vi "Helium Test - Step 5.vi"(7 "Step":i32, 8 "error in":errorcluster, 9 "Test Results In":T9, 10 "Gas":T8, 11 "Test Configuration":T1) -> (0 "error out":errorcluster, 1 "Test Results Out":T9, 2 "Gas Out":T8 caption="Gas", 3 "Test Configuration Out":T1)   [LabVIEW 2015]
uses:
  CAN Communication/PAS/Typedefs/Session Handle.ctl
  CAN Communication/PAS/PAS.lvclass
  Controls/Test Results.ctl
  Controls/Step Result.ctl
  Controls/Test Configuration.ctl
  Controls/Vacuum Test.ctl
  Controls/Test Timing.ctl
  Controls/Vaccum Thresholds.ctl
  Controls/Helium Test.ctl
  Controls/Helium Thresholds.ctl
  Controls/Functional Test.ctl
  CAN Communication/PAS/Typedefs/Valves.ctl
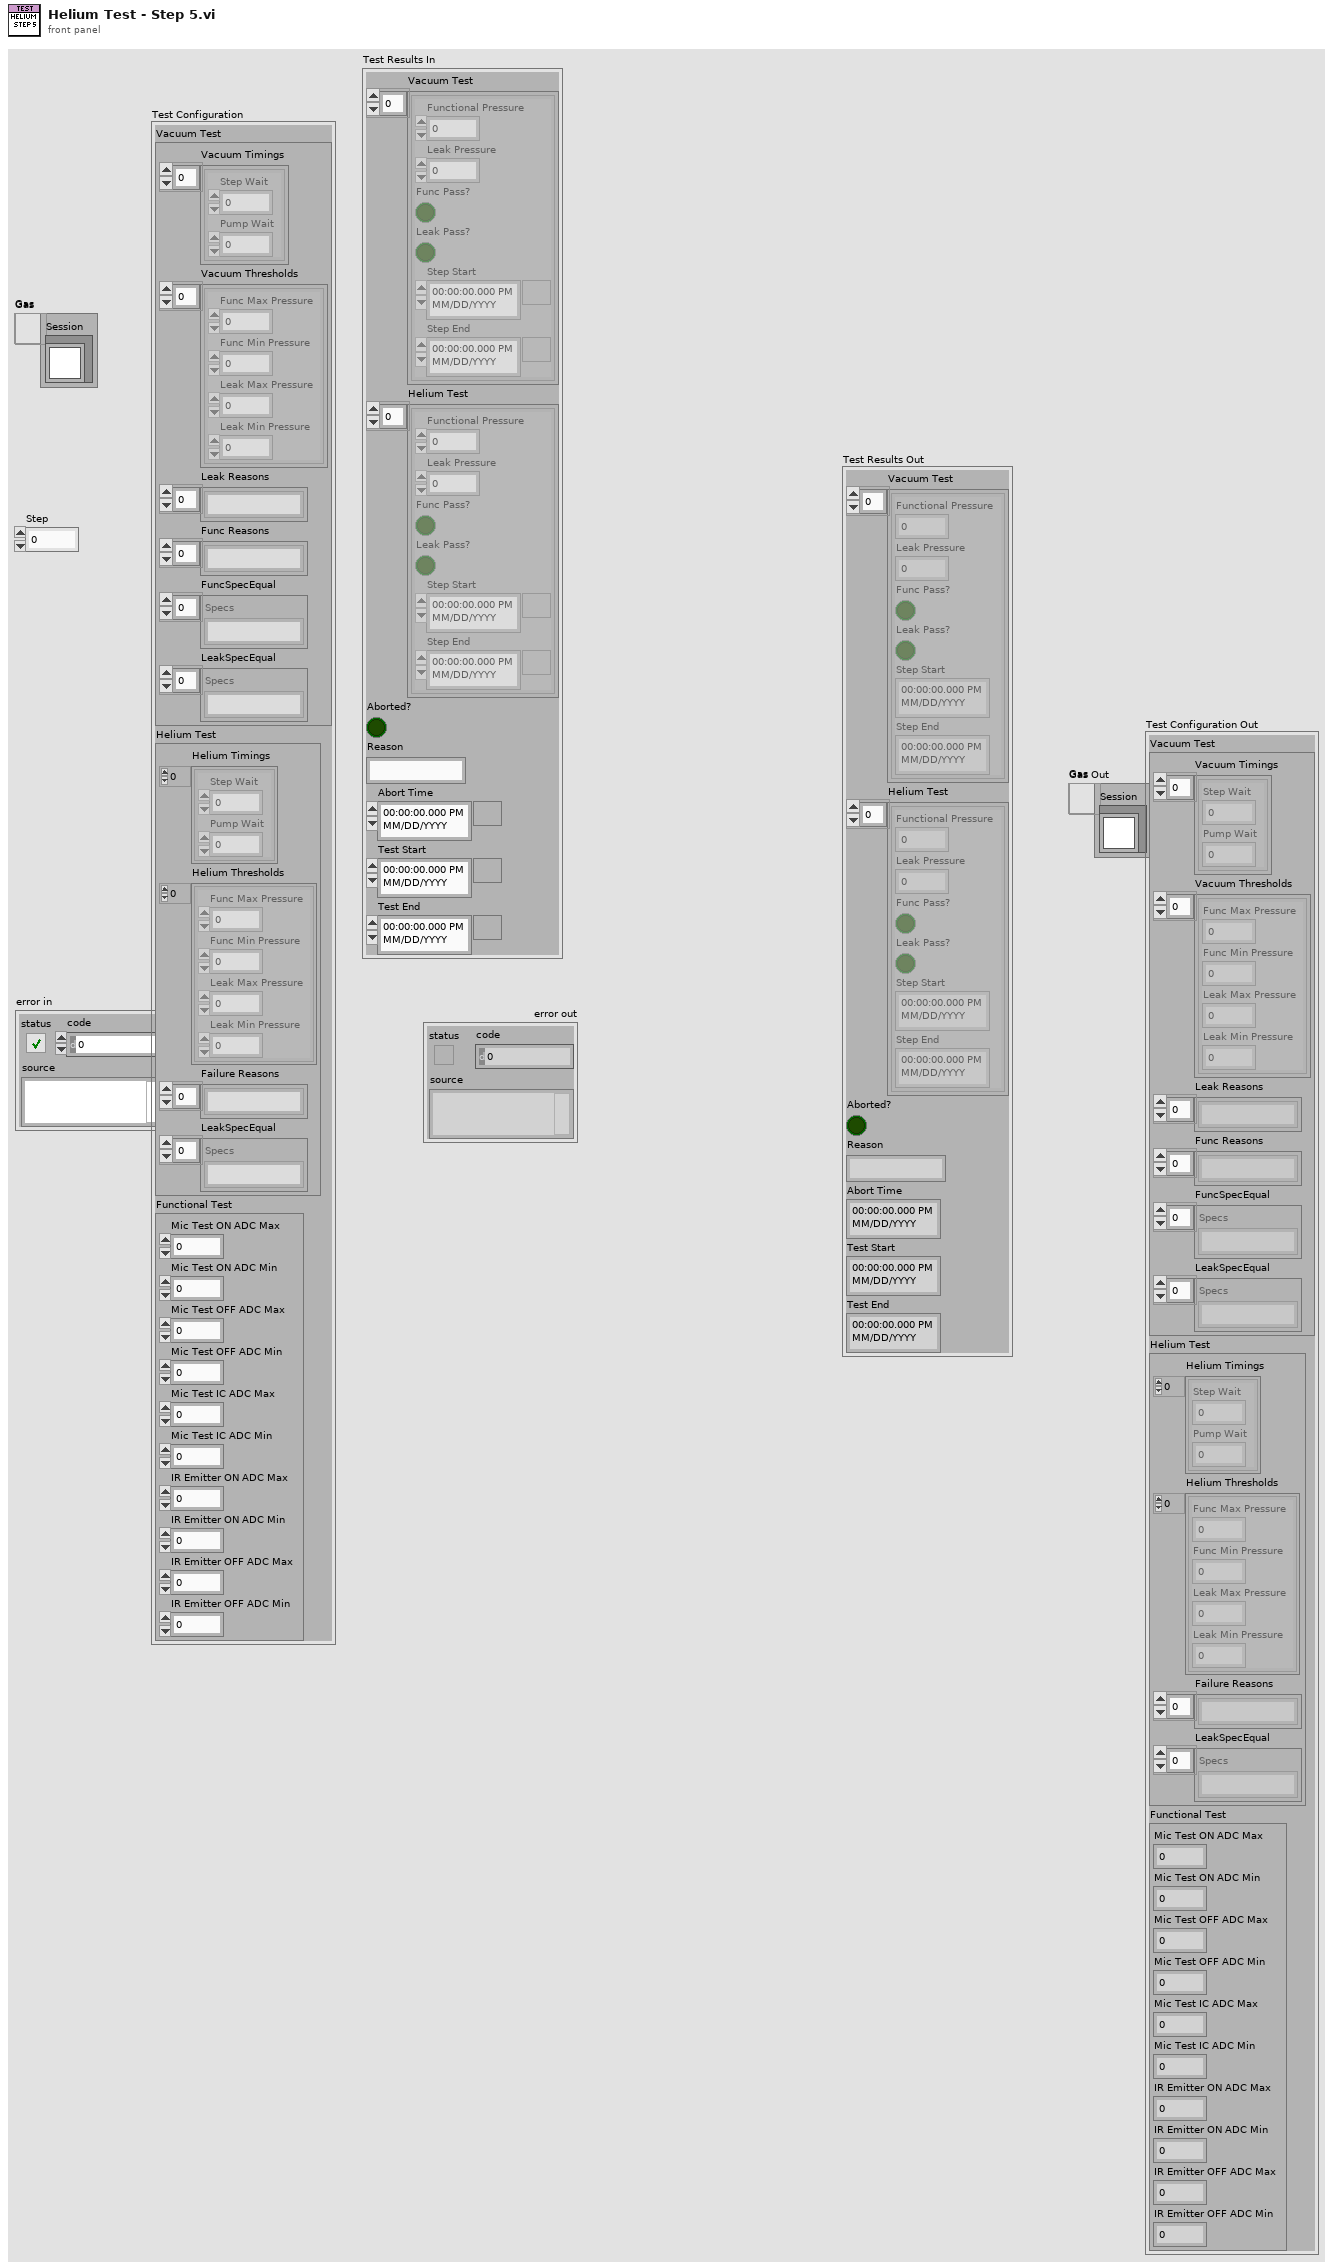
[diagram p1: front panel]
types:
  T1 = typedef "Test Configuration.ctl" = cluster{"Vacuum Test":T2, "Helium Test":T5, "Functional Test":T7}
  T2 = typedef "Vacuum Test.ctl" = cluster{"Vacuum Timings":T3[], "Vacuum Thresholds":T4[], "Leak Reasons":string[], "Func Reasons":string[], "FuncSpecEqual":string[], "LeakSpecEqual":string[]}
  T3 = typedef "Test Timing.ctl" = cluster{"Step Wait":dbl, "Pump Wait":dbl}
  T4 = typedef "Vaccum Thresholds.ctl" = cluster{"Func Max Pressure":dbl, "Func Min Pressure":dbl, "Leak Max Pressure":dbl, "Leak Min Pressure":dbl}
  T5 = typedef "Helium Test.ctl" = cluster{"Helium Timings":T3[], "Helium Thresholds":T6[], "Failure Reasons":string[], "LeakSpecEqual":string[]}
  T6 = typedef "Helium Thresholds.ctl" = cluster{"Func Max Pressure":dbl, "Func Min Pressure":dbl, "Leak Max Pressure":dbl, "Leak Min Pressure":dbl}
  T7 = typedef "Functional Test.ctl" = cluster{"Mic Test ON ADC Max":dbl, "Mic Test ON ADC Min":dbl, "Mic Test OFF ADC Max":dbl, "Mic Test OFF ADC Min":dbl, "Mic Test IC ADC Max":dbl, "Mic Test IC ADC Min":dbl, "IR Emitter ON ADC Max":dbl, "IR Emitter ON ADC Min":dbl, "IR Emitter OFF ADC Max":dbl, "IR Emitter OFF ADC Min":dbl}
  T8 = typedef "PAS.lvclass/Session Handle.ctl" = refnum<data-value>
  T9 = typedef "Test Results.ctl" = cluster{"Vacuum Test":T10[], "Helium Test":T10[], "Aborted?":bool, "Reason":string, "Abort Time":timestamp, "Test Start":timestamp, "Test End":timestamp}
  T10 = typedef "Step Result.ctl" = cluster{"Functional Pressure":dbl, "Leak Pressure":dbl, "Func Pass?":bool, "Leak Pass?":bool, "Step Start":timestamp, "Step End":timestamp}
  T11 = typedef "PAS.lvclass/Valves.ctl" = u16
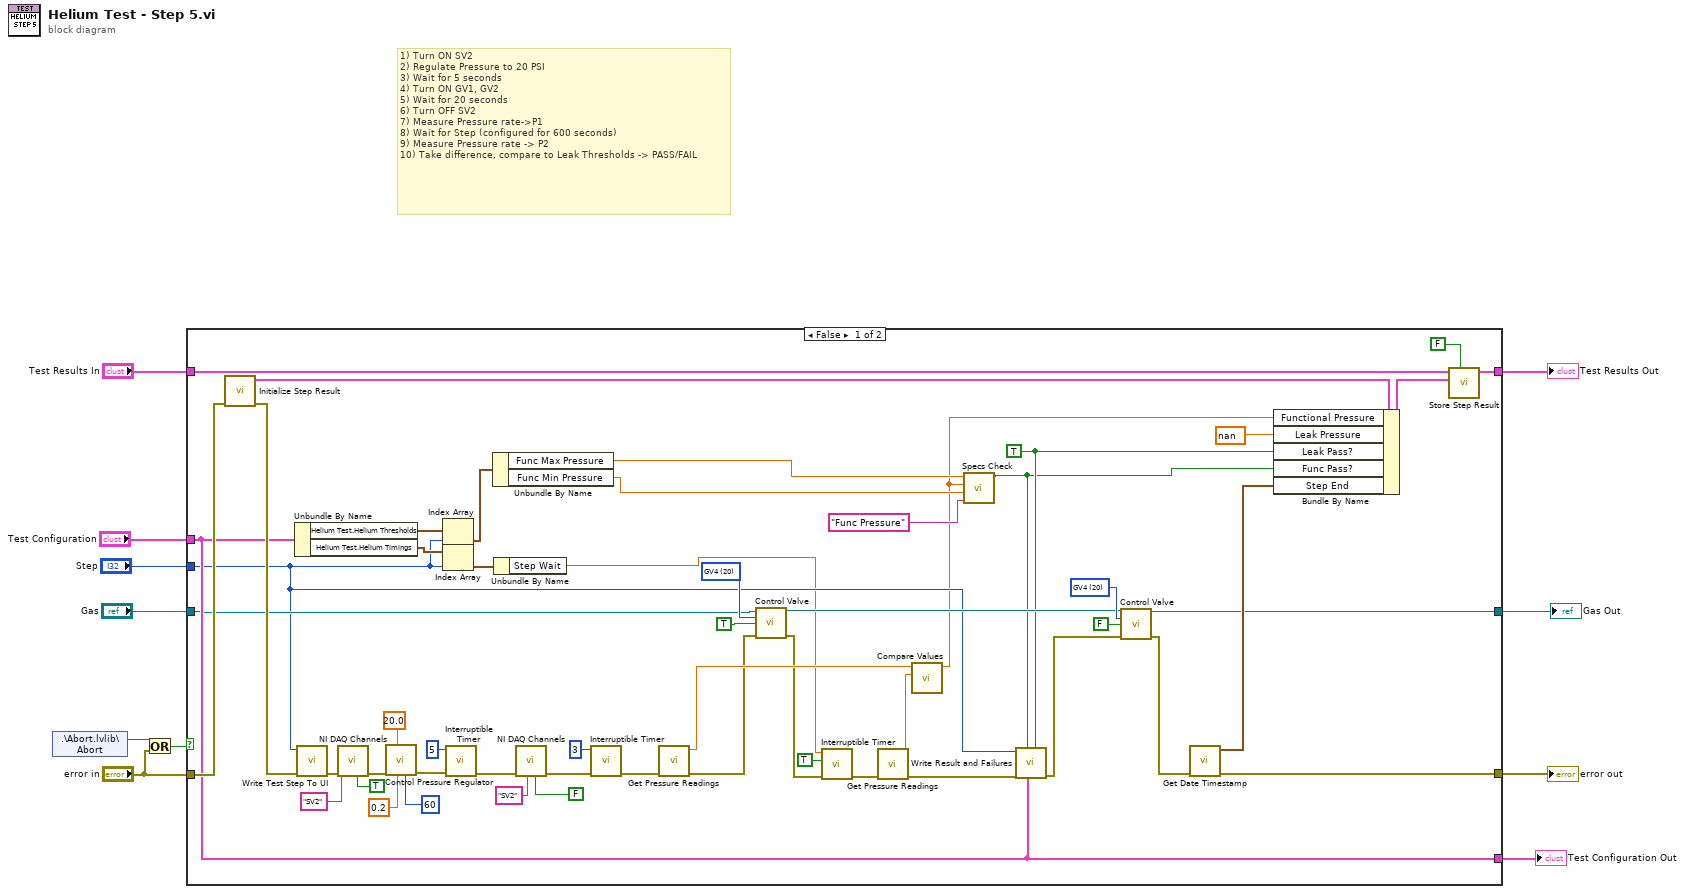
[diagram p0: block diagram]
diagram:
  # "1) Turn ON SV2\n2) Regulate Pressure to 20 PSI\n3) Wait for 5 seconds\n4) Turn ON GV1, GV2\n5) Wait for 20 seconds\n6) Turn OFF SV2\n7) Measure Pressure rate->P1\n8) Wait for Step (configured for 600 seconds)\n9) Measure Pressure rate -> P2\n10) Take difference, compare to Leak Thresholds -> PASS/FAIL"
  n1 = shared-variable ".\\Abort.lvlib\\Abort"() -> (w10:bool)  [unwired: 1 in, 1 out]
  n2 = Or(x=w10, y="error in") -> (x .or. y?=w9:bool)
  n3 = case shown="False" w9 {
    tunnel: "error in" -> [w65 w68]
    tunnel: "Test Results In" -> [w62 w69]
    tunnel: [w63 w69] -> w7
    tunnel: [w38 w68] -> w6
    tunnel: "Test Configuration" -> [w54 w67]
    tunnel: "Step" -> [w21 _]
    tunnel: [w54 w67] -> w1
    tunnel: [w43 w66] -> w3
    tunnel: "Gas" -> [w28 w66]
    frame False {
      w29 = T11 20 items=["GV1"=17, "GV2"=18, "GV3"=19, "GV4"=20] ("Valves")
      w20 = TRUE ("Update UI?")
      w44 = T11 20 items=["GV1"=17, "GV2"=18, "GV3"=19, "GV4"=20] ("Valves")
      n4 = call "Initialize Step Result.vi"("error in (no error)"=w65) -> ("error out"=w64:errorcluster, "New Step Result"=w61:T10)  [unwired: 8 in, 1 out]
      n5 = Unbundle By Name(w54) -> ("Helium Test.Helium Thresholds"=w58:T6[], "Helium Test.Helium Timings"=w57:T3[])
      n6 = call "Write Test Step To UI.vi"("error in (no error)"=w64, "Step"=w21) -> ("error out"=w47:errorcluster)  [unwired: 9 in]
      n7 = call "NI DAQ Channels.vi"("Control"=TRUE ("State"), "Channel"="SV2", "error in (no error)"=w47) -> ("error out"=w50:errorcluster)  [unwired: 7 in, 1 out]
      n8 = call "Control Pressure Regulator.vi"("Timeout"=60, "y"=0.2, "error in"=w50, "Desired PSI"=20.0) -> ("error out"=w48:errorcluster)  [unwired: 6 in, 1 out]
      n9 = Index Array(array=w58, index=w21) -> (element=w55:T6)
      n10 = Index Array(array=w57, index=w21) -> (element=w56:T3)
      n11 = call "Interruptible Timer.vi"("error in (no error)"=w48, "Wait (s)"=5) -> ("error out"=w35:errorcluster)  [unwired: 7 in, 2 out]
      n12 = Unbundle By Name(w55) -> ("Func Max Pressure"=w17:dbl, "Func Min Pressure"=w16:dbl)
      n13 = Unbundle By Name(w56) -> ("Step Wait"=w13:dbl)
      n14 = call "NI DAQ Channels.vi"("Control"=FALSE ("State"), "Channel"="SV2", "error in (no error)"=w35) -> ("error out"=w34:errorcluster)  [unwired: 7 in, 1 out]
      n15 = call "Interruptible Timer.vi"("error in (no error)"=w34, "Wait (s)"=3) -> ("error out"=w32:errorcluster)  [unwired: 7 in, 2 out]
      n16 = call "Get Pressure Readings.vi"("error in (no error)"=w32) -> ("error out"=w26:errorcluster, "NI-DAQ Pressure"=w31:dbl)  [unwired: 7 in, 2 out]
      n17 = call "Control Valve.vi"("Session Handle in"=w28, "Valves"=w29, "Energize?"=TRUE ("State"), "error in (no error)"=w26) -> ("Session Handle out"=w27:T8, "error out"=w25:errorcluster)  [unwired: 8 in, 2 out]
      n18 = call "Interruptible Timer.vi"("error in (no error)"=w25, "Update UI?"=TRUE, "Wait (s)"=w13) -> ("error out"=w24:errorcluster)  [unwired: 6 in, 2 out]
      n19 = call "Get Pressure Readings.vi"("error in (no error)"=w24) -> ("error out"=w23:errorcluster, "NI-DAQ Pressure"=w22:dbl)  [unwired: 7 in, 2 out]
      n20 = call "Compare Values.vi"("P2"=w22, "P1"=w31) -> ("Abs Diff"=w14:dbl)  [unwired: 9 in]
      n21 = call "Specs Check.vi"("parameter"="Func Pressure", "lower limit"=w16, "x"=w14, "upper limit"=w17) -> ("In Range?"=w18:bool)  [unwired: 6 in, 1 out]
      n22 = call "Write Result and Failures.vi"("Leak"=w20, "Test Configuration"=w54, "Func"=w18, "error in (no error)"=w23, "Step"=w21) -> ("error out"=w39:errorcluster)  [unwired: 6 in]
      n23 = call "Control Valve.vi"("Session Handle in"=w27, "Valves"=w44, "Energize?"=FALSE, "error in (no error)"=w39) -> ("Session Handle out"=w43:T8, "error out"=w42:errorcluster)  [unwired: 8 in, 2 out]
      n24 = call "Get Date Timestamp.vi"("error in (no error)"=w42) -> ("error out"=w38:errorcluster, "current time"=w59:timestamp)  [unwired: 9 in]
      n25 = Bundle By Name(cluster=w61, "Functional Pressure"=w14, "Leak Pressure"=nan ("Functional Pressure"), "Leak Pass?"=w20, "Func Pass?"=w18, "Step End"=w59) -> (w60:T10)
      n26 = call "Store Step Result.vi"("Vacuum?"=FALSE, "Step Result"=w60, "Test Results In"=w62) -> ("Test Results Out"=w63:T9)  [unwired: 8 in]
    }
    frame True {
    }
  }
  "error out" <- w6
  "Test Results Out" <- w7
  "Gas Out" <- w3
  "Test Configuration Out" <- w1
